vi "CRC-16.vi"(11 "String in":string) -> (1 "CRC-16":u8=105, 2 "CRC-16 2":string="Mi", 3 "String out":string)   [LabVIEW 2019]
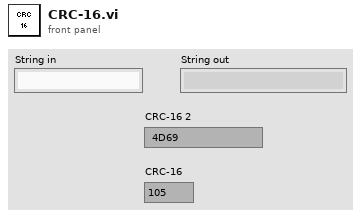
[diagram p1: front panel]
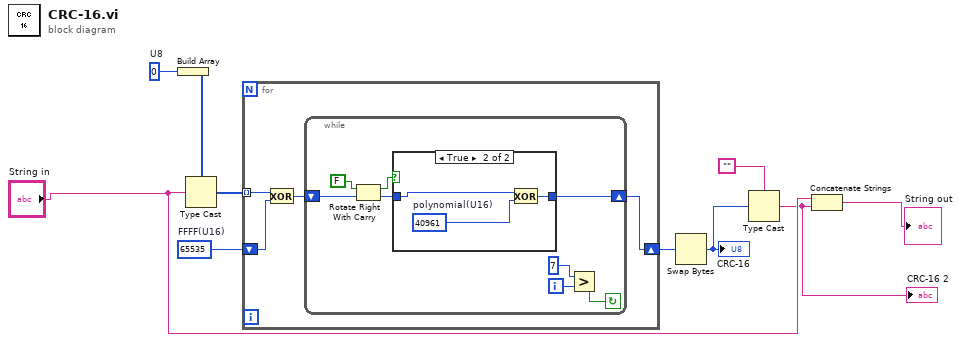
[diagram p0: block diagram]
diagram:
  w7 = u16 65535  # FFFF(U16)
  w1 = u8 0  # U8
  n1 = Build Array(w1) -> (w2:u8[])
  n2 = Type Cast(type=w2, x="String in") -> (*(type *) &x=w3:u8[])
  n3 = for {
    tunnel: w3 -> [w14] mode=indexing
    shift-right: [w11] -> w8
    shift-left: w7 -> [w13]
    n4 = Exclusive Or(1:w13, 2:w14) -> (0:w12:u16)
    n5 = while {
      shift-right: [w18] -> w11
      shift-left: w12 -> [w16]
      i -> [w17]
      stop <- w15 continue-if-true
      n6 = Rotate Right With Carry(2:w16, 3:FALSE) -> (0:w19:u16, 1:w20:bool)
      n7 = case shown="True" w20 {
        tunnel: w19 -> [w23 w26]
        tunnel: [w23 w24] -> w18
        frame False {
        }
        frame True {
          w25 = u16 40961  # polynomial(U16)
          n8 = Exclusive Or(1:w25, 2:w26) -> (0:w24:u16)
        }
      }
      n9 = Greater?(x=7, y=w17) -> (0:w15:bool)
    }
  }
  n10 = Swap Bytes(anything=w8) -> (byte swapped=w4:u16)
  "CRC-16" <- w4
  n11 = Type Cast(type="", x=w4) -> (*(type *) &x=w6:string)
  "CRC-16 2" <- w6
  n12 = Concatenate Strings("String in", w6) -> (→"String out":string)
